vi "Metadata tag number.vi"() -> (0 "Tag to store\nmetadata in\n(ImageID tag)":u16=32781)   [LabVIEW 2015, in "Tiff reader.lvlib"]
doc: "A constant that tells what tag number should be used for the metadata. (I have chosen 32781, the ImageID tag)"
uses:
  Tiff reader.lvlib
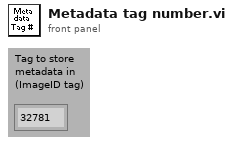
[diagram p1: front panel]
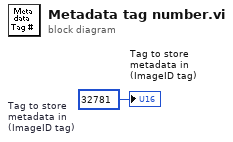
[diagram p0: block diagram]
diagram:
  w1 = u16 32781  # Tag to store metadata in (ImageID tag)
  "Tag to store\nmetadata in\n(ImageID tag)" <- w1
